vi "Read Selection.vi"(8 "error in (no error)":errorcluster, 11 "TreeSelection in":refnum<class "TreeSelection.lvclass">) -> (0 "error out":errorcluster, 2 "Selection[]":string[](array[string]), 3 "TreeSelection out":refnum<class "TreeSelection.lvclass">)   [LabVIEW 2015, in "TreeSelection.lvclass"]
doc: "This property gets or sets the items which are selected (have the TRUE checkbox).\n<b> </b> <b> </b>\n©2016 Q Software Innovations, LLC (QSI)\nwritten by Quentin Alldredge\nproduced in LabVIEW 2015\n\nsupport@qsoftwareinnovations.com\nwww.qsoftwareinnovations.com\n\nAll rights reserved.\n\nRedistribution and use in source and binary forms, with or without modification, are permitted provided that the following conditions are met:\n\n * Redistributions of source code must retain the above copyright notice, this list of conditions and the following disclaimer.\n * Redistributions in binary form must reproduce the above copyright notice, this list of conditions and the following disclaimer in the documentation and/or other materials provided with the distribution.\n * Neither the name of Q Software Innovations, LLC. nor the names of its contributors may be used to endorse or promote products derived from this software without specific prior written permission.\n\nTHIS SOFTWARE IS PROVIDED BY THE COPYRIGHT HOLDERS AND CONTRIBUTORS \"AS IS\" AND ANY EXPRESS OR IMPLIED WARRANTIES, INCLUDING, BUT NOT LIMITED TO, THE IMPLIED WARRANTIES OF MERCHANTABILITY AND FITNESS FOR A PARTICULAR PURPOSE ARE DISCLAIMED. IN NO EVENT SHALL THE COPYRIGHT OWNER OR CONTRIBUTORS BE LIABLE FOR ANY DIRECT, INDIRECT, INCIDENTAL, SPECIAL, EXEMPLARY, OR CONSEQUENTIAL DAMAGES (INCLUDING, BUT NOT LIMITED TO, PROCUREMENT OF SUBSTITUTE GOODS OR SERVICES; LOSS OF USE, DATA, OR PROFITS; OR BUSINESS INTERRUPTION) HOWEVER CAUSED AND ON ANY THEORY OF LIABILITY, WHETHER IN CONTRACT, STRICT LIABILITY, OR TORT (INCLUDING NEGLIGENCE OR OTHERWISE) ARISING IN ANY WAY OUT OF THE USE OF THIS SOFTWARE, EVEN IF ADVISED OF THE POSSIBILITY OF SUCH DAMAGE."
uses:
  TreeSelection.lvclass
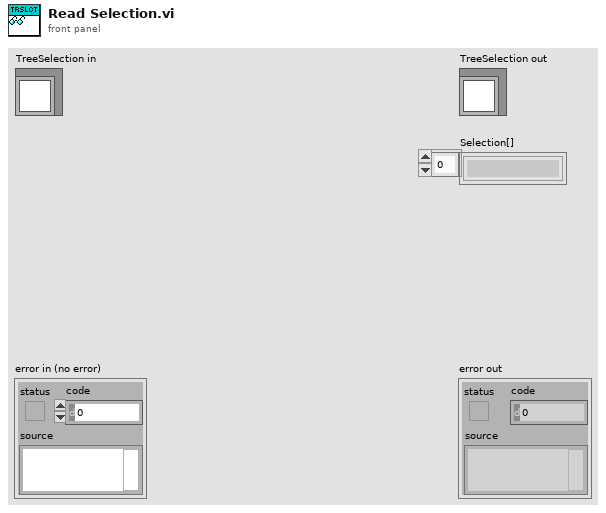
[diagram p1: front panel]
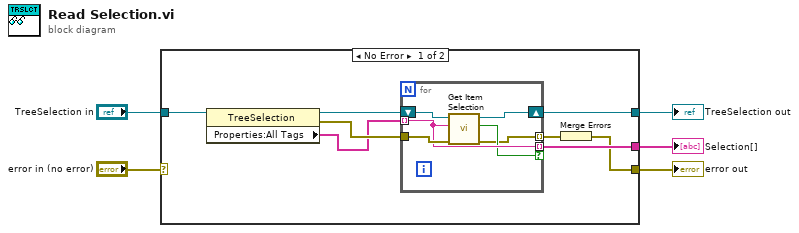
[diagram p0: block diagram]
diagram:
  n1 = case shown="No Error" "error in (no error)" {
    selector: "error in (no error)" -> [_ w21]
    tunnel: [w8 w21] -> w4
    tunnel: [w12 w20] -> w2
    tunnel: "TreeSelection in" -> [w13 w20]
    tunnel: [w10 _] -> w1
    frame No Error {
      n2 = property class="TreeSelection"(reference=w13) -> (reference out=w7:refnum<class "TreeSelection.lvclass">, error out=w11:errorcluster, "Properties:All Tags"=w6:string[])  [unwired: 1 in]
      n3 = for {
        shift-right: [w18] -> w12
        shift-left: w7 -> [w19]
        tunnel: w6 -> [w16] mode=indexing
        tunnel: w11 -> [w17]
        tunnel: [w16] -> w10 mode=indexing if=w15
        tunnel: [w14] -> w9 mode=indexing
        n4 = call "Get Item Selection.vi"("error in (no error)"=w17, "Tag"=w16, "TreeSelection in"=w19) -> ("error out"=w14:errorcluster, "IsSelected?"=w15:bool, "TreeSelection out"=w18:refnum<class "TreeSelection.lvclass">)  [unwired: 6 in]
      }
      n5 = Merge Errors(w9) -> (w8:errorcluster)
    }
    frame Error {
    }
  }
  "error out" <- w4
  "TreeSelection out" <- w2
  "Selection[]" <- w1
